vi "Consumer.vi"(8 "error in (no error)":errorcluster, 9 "Data":variant, 10 "Case ID":string, 11 "uService Template in":refnum<class "New uService Template.lvclass">) -> (0 "error out":errorcluster, 3 "uService Template out":refnum<class "New uService Template.lvclass">)   [LabVIEW 2020, in "New uService Template.lvlib" / "New uService Template.lvclass"]
uses:
  New uService Template.lvclass
  Consumer Case Selector.ctl
  TALOS/TALOS_PPL.lvlibp/Father of all uServices/Father of all uServices/Father of all uServices.lvclass
  New uService Template.lvclass/New uService Template.ctl
  TALOS/TALOS_PPL.lvlibp
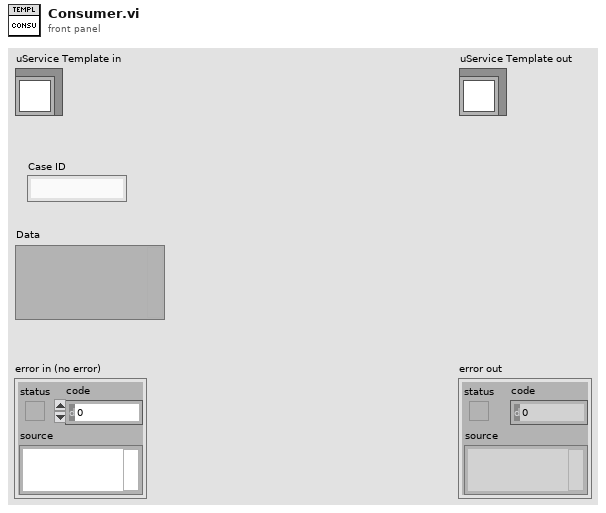
[diagram p1: front panel]
types:
  T1 = typedef "New uService Template.lvlib/New uService Template.lvclass/Consumer Case Selector.ctl" = enum16{"Example"}
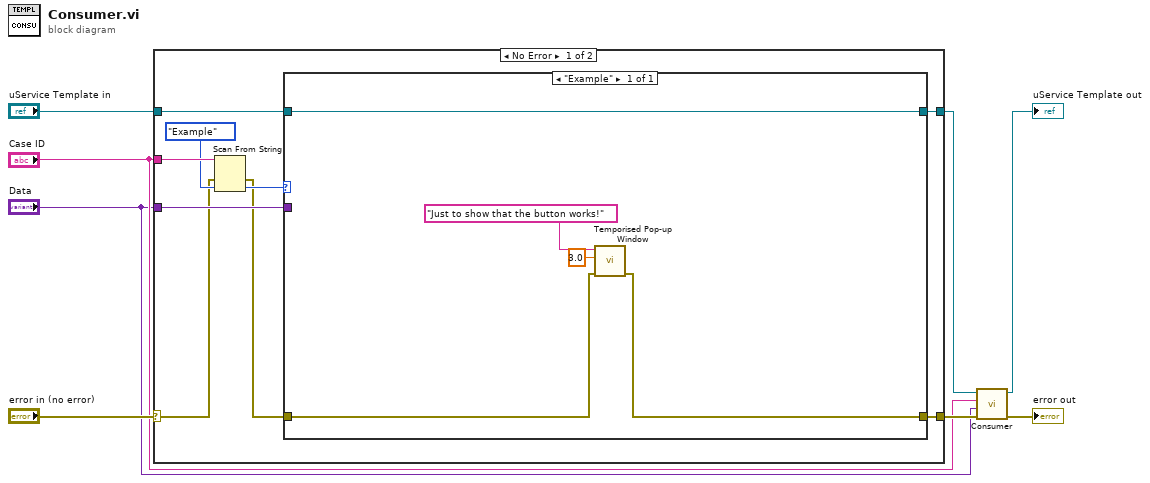
[diagram p0: block diagram]
diagram:
  n1 = case shown="No Error" "error in (no error)" {
    selector: "error in (no error)" -> [w10 w23]
    tunnel: [w16 w24] -> w3
    tunnel: "uService Template in" -> [w17 w24]
    tunnel: [w14 w23] -> w6
    tunnel: "Case ID" -> [w13 _]
    tunnel: "Data" -> [w15 _]
    frame No Error {
      n2 = Scan From String(input string=w13, error in=w10, default 1=Consumer_Case_Selector."Example" ("Consumer Case Selector")) -> (error out=w9:errorcluster, output 1=w11:T1)  [unwired: 2 in, 2 out]
      n3 = case shown="\"Example\"" w11 {
        tunnel: w17 -> [w22]
        tunnel: [w22] -> w16
        tunnel: w15 -> [_]
        tunnel: [w19] -> w14
        tunnel: w9 -> [w18]
        frame "Example" {
          n4 = call "Temporised Pop-up Window.vi"("error in (no error)"=w18, "Timeout"=3.0, "Text"="Just to show that the button works!" ("message")) -> ("error out"=w19:errorcluster)  [unwired: 8 in]
        }
      }
    }
    frame Error {
    }
  }
  n5 = call-parent "Consumer.vi"("error in (no error)"=w6, "Data"="Data", "Case ID"="Case ID", "uService Template in"=w3) -> ("error out"=→"error out":errorcluster, "uService Template out"=→"uService Template out":refnum<class "New uService Template.lvclass">)  [unwired: 6 in]
